vi "API.vi"(8 "error in (no error)":errorcluster, 11 "DataHandlerTask in":refnum<class "DataHandlerTask.lvclass">) -> (0 "error out":errorcluster, 2 "API":refnum<class "API.lvclass">, 3 "DataHandlerTask out":refnum<class "DataHandlerTask.lvclass">)   [LabVIEW 2020, in "VolatusData.lvlib" / "DataHandlerTask.lvclass"]
uses:
  DataHandlerTask.lvclass
  DataHandlerAPI/DataHandlerAPI.lvclass
  <vilib>/ActorFramework/Actor/Actor.lvclass
  C:/dev/lv20CE/relink/lv-volatus/Volatus/Task/Task.lvclass
  C:/Program Files (x86)/National Instruments/LabVIEW 2020/vi.lib/ActorFramework/Actor/Actor.lvclass
  C:/dev/lv20CE/relink/lv-volatus/Volatus/TaskStateHandler/TaskStateHandler.lvclass
  C:/dev/lv20CE/relink/lv-volatus/Volatus/VectoMessageHandler/VectoMessageHandler.lvclass
  C:/dev/lv20CE/relink/lv-volatus/Volatus/DataHandlerTask/DataHandlerTask.lvclass
  C:/dev/lv20CE/relink/lv-volatus/Volatus/API Provider/API Provider.lvclass
  C:/dev/lv20CE/relink/lv-volatus/Volatus/DataHandler/DataHandler.lvclass
  C:/dev/lv20CE/relink/lv-volatus/Volatus/DataHandlerAPI/DataHandlerAPI.lvclass
  C:/dev/lv20CE/relink/lv-volatus/Volatus/API/API.lvclass
  Volatus/API/API.lvclass
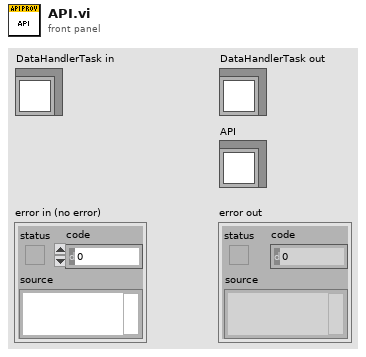
[diagram p1: front panel]
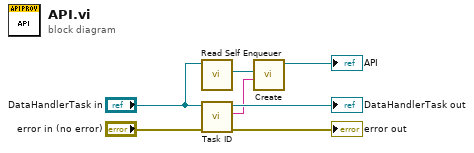
[diagram p0: block diagram]
diagram:
  n1 = call <vilib>:"Read Self Enqueuer.vi"("Actor"="DataHandlerTask in") -> ("Self Enqueuer"=w6:refnum<class "Message Enqueuer.lvclass">)  [unwired: 10 in]
  n2 = call-dynamic "Task ID.vi"("error in (no error)"="error in (no error)", "DataHandlerTask in"="DataHandlerTask in") -> ("error out"=→"error out":errorcluster, "Task ID"=w1:string, "DataHandlerTask out"=→"DataHandlerTask out":refnum<class "DataHandlerTask.lvclass">)  [unwired: 7 in]
  n3 = call "Create.vi"("Task ID"=w1, "EnQr"=w6) -> ("DataHandlerAPI out"=→"API":refnum<class "DataHandlerAPI.lvclass">)  [unwired: 8 in, 1 out]
